vi "Substitute Actor.vi"(10 "Substitute Actor in":refnum<class "Actor.lvclass">, 11 "Current Command States":refnum<class "Command States.lvclass">) -> (0 "error out":errorcluster, 2 "Substitute Actor out":refnum<class "Actor.lvclass">)   [LabVIEW 2013, in "Command Actor.lvlib" / "Command States.lvclass"]
doc: "(<B>Filename</B>: Actor Framework.lvlib:Actor.lvclass:Substitute Actor.vi)\n\nThis method copies information from the <b>Current Actor</b> to the <b>Substitute Actor</b>, including the to-self and the to-caller queue references. The purpose of this function is to allow an actor to define a method that replaces itself with another actor, useful for implementing a State Pattern Actor. Child classes should override this method to copy any additional fields that they need from the current to the substitute.\n\nThis method may return error code 678010: Illegal substitution. Overrides of this method may choose to return this error if the new actor is not one that is an appropriate substitute for the current actor, for whatever standards of \"appropriate\" are chosen for the current actor. If returning an error, override VIs should return the unmodified <b>Current Actor</b> as <b>Substitute Actor out</b>."
uses:
  Command States.lvclass
  <vilib>/ActorFramework/Actor/Actor.lvclass
  <vilib>/ni/Actors/State Actor/State Actor/State Actor.lvclass
  Command States.lvclass/Command States.ctl
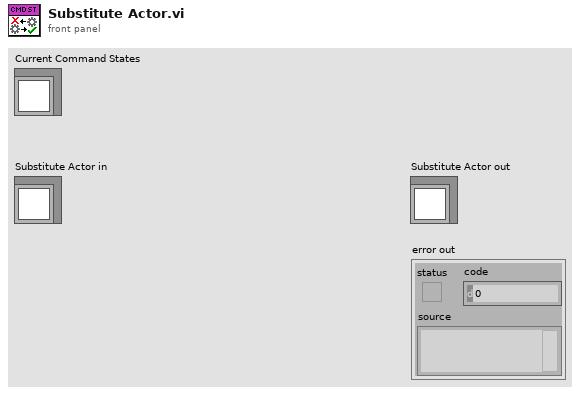
[diagram p1: front panel]
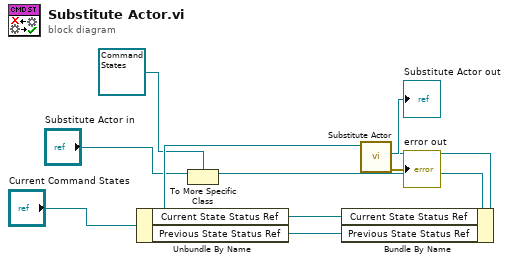
[diagram p0: block diagram]
diagram:
  n1 = Unbundle By Name("Current Command States") -> ("Current State Status Ref"=w2:refnum<vi>, "Previous State Status Ref"=w1:refnum<vi>)
  n2 = To More Specific Class(target class=refnum<class "Command States.lvclass"> refnum ("Command Actor.lvlib:Command States.lvclass"), reference="Substitute Actor in") -> (specific class reference=w4:refnum<class "Command States.lvclass">)  [unwired: 1 in, 1 out]
  n3 = Bundle By Name(cluster=w4, "Current State Status Ref"=w2, "Previous State Status Ref"=w1) -> (w3:refnum<class "Command States.lvclass">)
  n4 = call-parent "Substitute Actor.vi"("Substitute Actor in"=w3, "Current Actor"="Current Command States") -> ("error out"=→"error out":errorcluster, "Substitute Actor out"=→"Substitute Actor out":refnum<class "Actor.lvclass">)  [unwired: 8 in]
